vi "Deterministic Errors.To String.U8.vi"(11 "value":u8) -> (3 "value as string":string)   [LabVIEW 2016, in "Deterministic Error Builder.lvlib"]
uses:
  Deterministic Error Builder.lvlib
  Deterministic Errors.New Allocated String (16B).vi
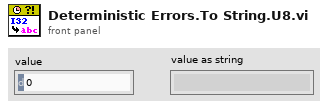
[diagram p1: front panel]
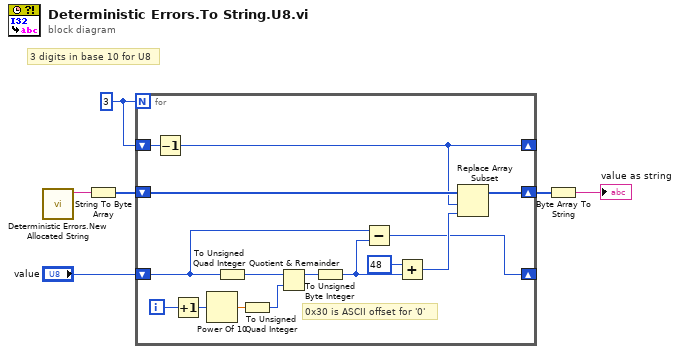
[diagram p0: block diagram]
diagram:
  w3 = 3
  # "3 digits in base 10 for U8"
  n1 = call-poly "Deterministic Errors.New Allocated String.vi"() -> ("16-byte string"=w2:string)  [unwired: 11 in]
  n2 = String To Byte Array(string=w2) -> (unsigned byte array=w4:u8[])
  n3 = for {
    N: w3 -> [_]
    shift-right: [w19] -> w6
    shift-left: w4 -> [w21]
    shift-right: [w14] -> _
    shift-left: w3 -> [w16]
    shift-right: [w7] -> _
    shift-left: "value" -> [w9]
    i -> [w13]
    # "0x30 is ASCII offset for '0'"
    n4 = Decrement(x=w16) -> (x-1=w14:i32)
    n5 = Increment(x=w13) -> (x+1=w12:i32)
    n6 = Power Of 10(x=w12) -> (10^x=w18:dbl)
    n7 = To Unsigned Quad Integer(1:w9) -> (0:w10:u64)
    n8 = To Unsigned Quad Integer(1:w18) -> (0:w17:u64)
    n9 = Quotient & Remainder(x=w10, y=w17) -> (x-y*floor(x/y)=w11:u64)  [unwired: 1 out]
    n10 = To Unsigned Byte Integer(number=w11) -> (unsigned 8bit integer=w8:u8)
    n11 = Subtract(x=w9, y=w8) -> (x-y=w7:u8)
    n12 = Add(x=u8 48 ("y"), y=w8) -> (x+y=w20:u8)
    n13 = Replace Array Subset(array=w21, new element=w20, index=w14) -> (w19:u8[])
  }
  n14 = Byte Array To String(unsigned byte array=w6) -> (string=→"value as string":string)
